vi "Read :: Write Shell Test.vi"() -> ()   [LabVIEW 2014]
panel:
  in  "Waveform index for Write":i32
  out "WaveformData Write":T1
  out "Waveform Graph Write":waveform(dbl)(graph)
  out "Waveform Graph":waveform(dbl)(graph)
  out "WaveformData":T1
  in  "stop":bool
  in  "Waveform index":i32
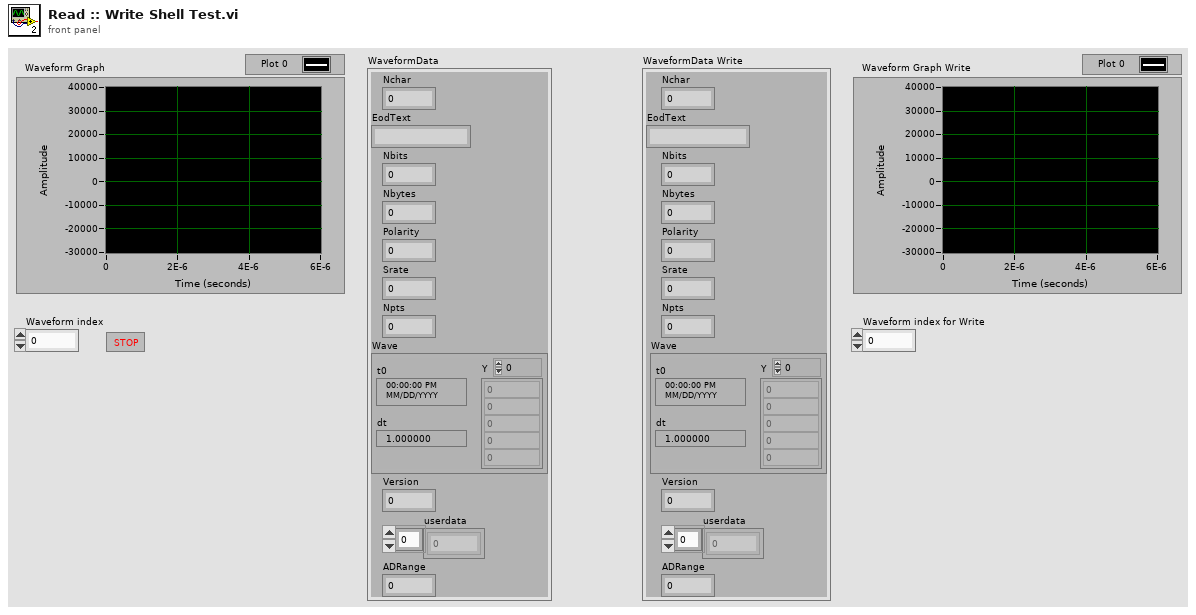
[diagram p1: front panel]
types:
  T1 = cluster{"Nchar":i32, "EodText":string, "Nbits":i32, "Nbytes":i32, "Polarity":i32, "Srate":i32, "Npts":i32, "Wave":waveform(dbl), "Version":i32, "userdata":dbl[], "ADRange":dbl}
  T2 = enum16{"open", "replace", "create", "open or create", "replace or create", "replace or create with confirmation"}
  T3 = cluster{"Nchar":i32, "EodText":string, "Nbits":i32, "Nbytes":i32, "Polarity":i32, "Srate":i32, "Npts":i32, "Wave":waveform(dbl), "Version":i32, "userdata":dbl[], "ADRange":dbl}[]
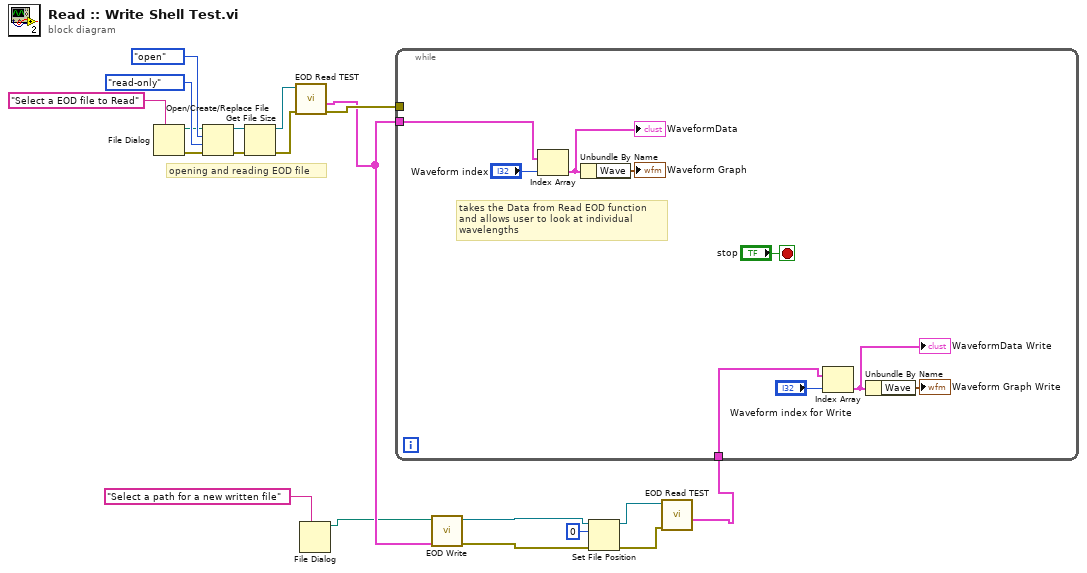
[diagram p0: block diagram]
diagram:
  # "opening and reading EOD file"
  n1 = File Dialog(7:"Select a EOD file to Read" ("prompt")) -> (0:w16:errorcluster, 3:w14:path)  [unwired: 6 in, 2 out]
  n2 = Open/Create/Replace File(file path (use dialog)=w14, error in=w16, operation (0:open)=T2."open", access (0:read/write)=enum16{"read/write", "read-only", "write-only"}."read-only") -> (refnum out=w19:refnum<file>, error out=w15:errorcluster)  [unwired: 2 in, 1 out]
  n3 = Get File Size(file=w19, error in=w15) -> (refnum out=w11:refnum<file>, 0:w10:errorcluster)  [unwired: 1 out]
  n4 = call "EOD Read TEST.vi"("error in (no error)"=w10, "Byte Stream File in"=w11) -> ("error out"=w12:errorcluster, "EODDataOut"=w6:T3)  [unwired: 6 in, 2 out]
  n5 = File Dialog(7:"Select a path for a new written file" ("prompt")) -> (3:w3:path)  [unwired: 6 in, 3 out]
  n6 = call "EOD Write.vi"("EODDataInput"=w6, "file path (use dialog)"=w3) -> ("error out"=w4:errorcluster, "refnum out"=w5:refnum<file>)  [unwired: 8 in]
  n7 = Set File Position(offset (in bytes) (0)=i64 0, refnum=w5, error in=w4) -> (refnum out=w9:refnum<file>, error out=w8:errorcluster)  [unwired: 1 in]
  n8 = call "EOD Read TEST.vi"("error in (no error)"=w8, "Byte Stream File in"=w9) -> ("EODDataOut"=w7:T3)  [unwired: 6 in, 3 out]
  n9 = while {
    tunnel: w6 -> [w24]
    tunnel: w12 -> [_]
    tunnel: w7 -> [w20]
    stop <- "stop" stop-if-true
    # "takes the Data from Read EOD function\nand allows user to look at individual\nwavelengths"
    n10 = Index Array(array=w24, index="Waveform index") -> (element=w25:T1)
    "WaveformData" <- w25
    n11 = Unbundle By Name(w25) -> ("Wave"=→"Waveform Graph":waveform(dbl))
    n12 = Index Array(array=w20, index="Waveform index for Write") -> (element=w21:T1)
    "WaveformData Write" <- w21
    n13 = Unbundle By Name(w21) -> ("Wave"=→"Waveform Graph Write":waveform(dbl))
  }
